vi "Controller Test Bench (17).vi"(5 "Folder to save file to":path=path "C:/Users/LAV-UFSC-2023/Documents/LAV-TCC/Dados-Experimentos/Dados-Bancada-LABVIEW", 6 "Signal Output\nControl":enum32{"White Noise", "Harmonic"}(tab), 7 "stop":bool, 8 "Enable Display":bool=TRUE, 9 "Accel. 2":bool, 10 "Output":bool=TRUE) -> (0 "New file path":path, 2 "Accel. 1 Raw":dbl[](graph), 3 "Output Signal":dynamicdata(graph))   [LabVIEW 2022 SP3]
uses:
  WhiteNoise.ctl
  <vilib>/Utility/error.llb/DialogType.ctl
  <vilib>/Platform/TimedLoop/XDataNode/timing_clust.ctl
  <vilib>/Platform/TimedLoop/XDataNode/nitl_modes.ctl
  <vilib>/Platform/TimedLoop/XDataNode/wakeup.ctl
  <vilib>/DAQmx/create/channels.llb/DAQmx Create Channel (AI-Acceleration-Accelerometer).vi
  <vilib>/DAQmx/configure/timing.llb/DAQmx Timing (Sample Clock).vi
  <vilib>/DAQmx/miscellaneous.llb/DAQmx Fill In Error Info.vi
  <vilib>/platform/TimedLoop/XDataNode/XDataNode.xnode
  <vilib>/DAQmx/read.llb/DAQmx Read (Analog 1D DBL 1Chan NSamp).vi
  <vilib>/DAQmx/write.llb/DAQmx Write (Analog 2D DBL NChan NSamp).vi
  <vilib>/DAQmx/create/channels.llb/DAQmx Create Channel (AO-Voltage-Basic).vi
  <vilib>/measure/NI_MABase.lvlib
  <vilib>/Platform/TimedLoop/XDataNode/XDNodeRunTimeDep.lvlib
panel:
  out "Frame 2 Duration":i64
  out "Frame 1 Duration":i64
  in  "White Noise\nParameters":T2={"Seed"=0.0, "Standard Deviation"=2.0, "Reset"=FALSE, "Iterator"=1.0, "Seed"=-1, "Lower Cut-Off"=5.0, "Upper Cut-Off"=350.0} {"Upper Cut-Off" min=5.0 max=350.0 step=10.0; "Lower Cut-Off" min=5.0 max=350.0 step=10.0; "Standard Deviation" min=0.001 max=3.0 step=0.05 format="%0.2p"}
  in  "Hamonic\nParameters":T3={"Waveform Type"=0, "Frequency"=10.0, "Amplitude"=0.25} {"Frequency" min=5.0 max=350.0 step=10.0 format="%0.2p"; "Waveform Type" items=["Sine Wave", "Triangle Wave", "Square Wave", "Sawtooth Wave"]; "Amplitude" min=0.001 max=0.3 step=0.05 format="%0.2p"}
  # "Filter"
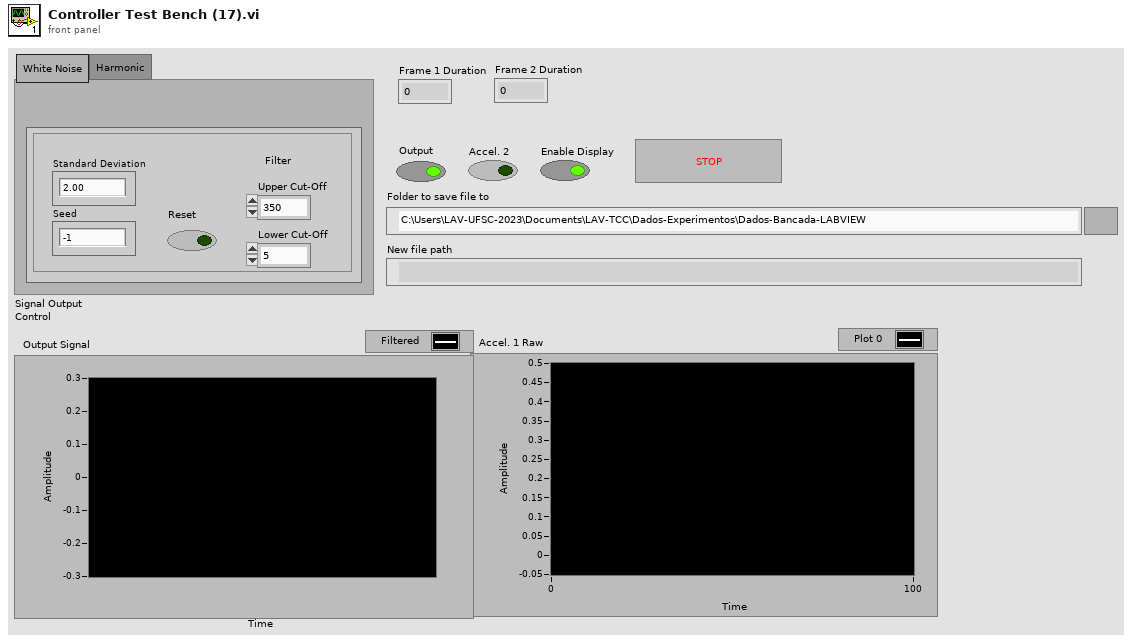
[diagram p1: front panel]
types:
  T1 = typedef "WhiteNoise.ctl" = dbl
  T2 = cluster{"Seed":T1, "Standard Deviation":dbl, "Reset":bool, "Iterator":dbl, "Seed":i8, "Lower Cut-Off":dbl, "Upper Cut-Off":dbl}
  T3 = cluster{"Waveform Type":u16, "Frequency":dbl, "Amplitude":dbl}
  T4 = typedef "DialogType.ctl" = u16
  T5 = enum16{"open", "open or create", "create or replace", "create", "open (read-only)"}
  T6 = typedef "XDNodeRunTimeDep.lvlib/timing_clust.ctl" = cluster{"Expected End [f-1]":u64, "Actual End [f-1]":u64, "Finished Late? [f-1]":bool, "Expected End [i-1]":u64, "Actual End [i-1]":u64, "Finished Late? [i-1]":bool, "Expected Start [i]":u64, "Actual Start [i]":u64, "Expected Start [f]":u64, "Actual Start [f]":u64, "Source Name":string, "Structure Name":string, "Period":i64, "Deadline":i64, "Offset":i64, "Start":i64, "Priority":i32, "Timeout":i32, "Mode":T7, "Wakeup Reason":T8, "Error":errorcluster, "Source Type":string, "Secondary Source Type":string, "Global End Time":u64, "Global Start Time":u64, "Frame Duration":u64, "Iteration Duration":u64, "Assigned CPU":i32, "I/O Scan Engine Mode":u32}
  T7 = typedef "XDNodeRunTimeDep.lvlib/nitl_modes.ctl" = enum32{"No Change", "Process missed periods, maintain original phase", "Discard missed periods, maintain original phase", "Process missed periods, ignore original phase", "Discard missed periods, ignore original phase"}
  T8 = typedef "XDNodeRunTimeDep.lvlib/wakeup.ctl" = enum32{"Normal", "Aborted", "Asynchronous wakeup", "Timing source error", "Timed loop error", "Timeout"}
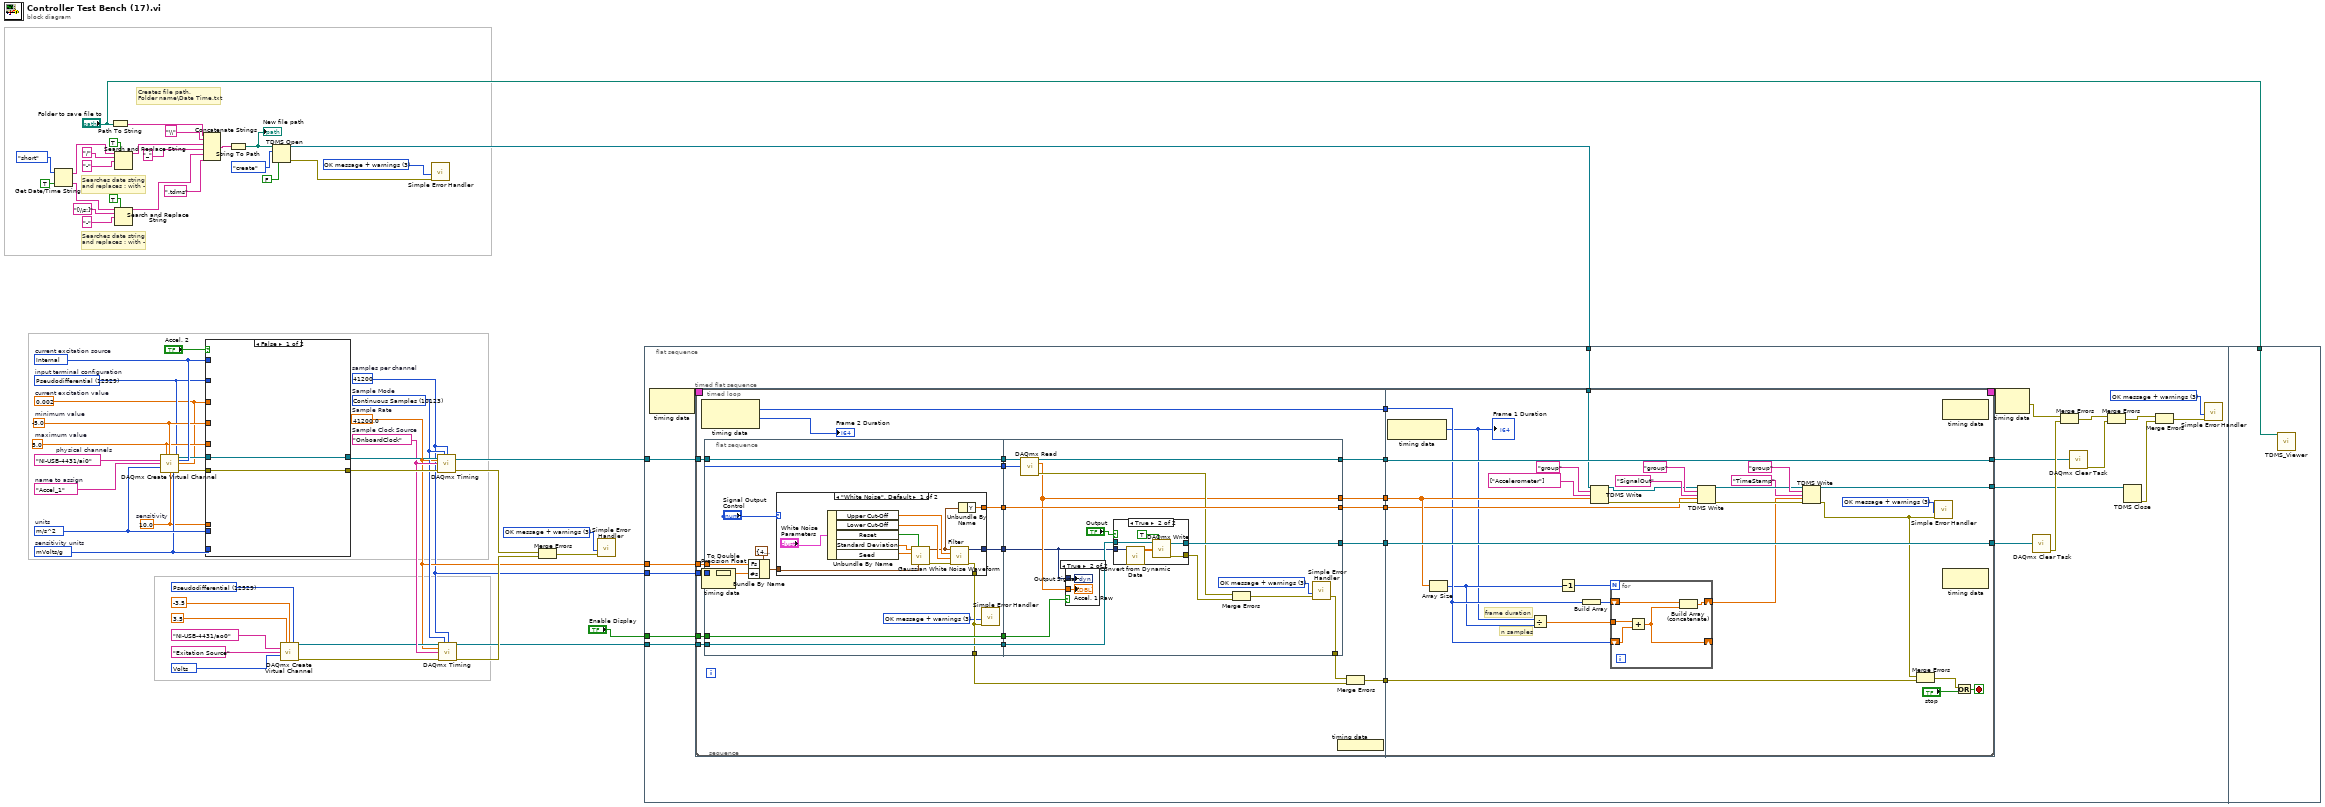
[diagram p0: block diagram]
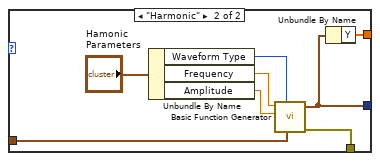
[diagram p2: hidden frame]
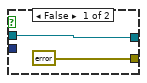
[diagram p4: hidden frame]
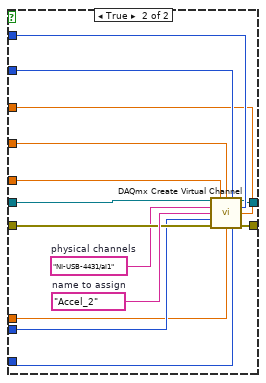
[diagram p5: hidden frame]
diagram:
  w10 = T4 3 items=["no dialog", "OK message", "continue or stop message", "OK message + warnings", "continue/stop + warnings"] ("type of dialog (OK msg:1)")
  w6 = 41200  # samples per channel
  w12 = T4 3 items=["no dialog", "OK message", "continue or stop message", "OK message + warnings", "continue/stop + warnings"] ("type of dialog (OK msg:1)")
  w45 = 12529 items=["Default"=-1, "RSE"=10083, "Differential"=10106, "Pseudodifferential"=12529] ("output terminal configuration")
  w43 = 10348 items=["Volts"=10348, "From Custom Scale"=10065] ("units")
  w49 = 12509 items=["mVolts/g"=12509, "Volts/g"=12510]  # sensitivity units
  w40 = 10.0  # sensitivity
  w48 = 0.002  # current excitation value
  w56 = 10200 items=["Internal"=10200, "External"=10167, "None"=10230]  # current excitation source
  w50 = tag "NI-USB-4431/ai0"  # physical channels
  w37 = tag "OnboardClock"  # Sample Clock Source
  w7 = 41200.0  # Sample Rate
  w36 = 10123 items=["Finite Samples"=10178, "Continuous Samples"=10123, "Hardware Timed Single Point"=12522]  # Sample Mode
  w52 = 12529 items=["default"=-1, "RSE"=10083, "NRSE"=10078, "Differential"=10106, "Pseudodifferential"=12529]  # input terminal configuration
  w55 = -5.0  # minimum value
  w54 = 5.0  # maximum value
  w58 = "Accel_1"  # name to assign
  w53 = 12470 items=["g"=10186, "m/s^2"=12470, "in/s^2"=12471, "From Custom Scale"=10065]  # units
  # "Searches date string\nand replaces : with -"
  # "Searches date string\nand replaces : with -"
  # "Creates file path.\nFolder name\\Date Time.txt"
  n1 = Get Date/Time String(date format (0)=enum16{"short", "long", "abbreviated"}."short", want seconds? (F)=TRUE) -> (date string=w15:string, time string=w28:string)  [unwired: 1 in]
  n2 = Path To String(path="Folder to save file to") -> (string=w23:string)
  n3 = Search and Replace String(replace all?=TRUE ("replace all? (F)"), input string=w15, search string="/" ("replace string (\"\")"), replace string="-" ("replace string (\"\")")) -> (result string=w14:string)  [unwired: 4 in, 3 out]
  n4 = Search and Replace String(replace all?=TRUE ("replace all? (F)"), input string=w28, search string="[\\s:]" ("replace string (\"\")"), replace string="-" ("replace string (\"\")")) -> (result string=w21:string)  [unwired: 4 in, 3 out]
  n5 = call-poly <vilib>:"DAQmx Create Virtual Channel.vi"("maximum value"=w54, "minimum value"=w55, "input terminal configuration"=w52, "physical channels"=w50, "current excitation source"=w56, "name to assign"=w58, "current excitation value"=w48, "units"=w53, "sensitivity"=w40, "sensitivity units"=w49) -> ("task out"=w51:refnum<k21>, "error out"=w57:errorcluster)  [unwired: 4 in]
  n6 = Concatenate Strings(w23, "\\" ("string"), w14, "_" ("string"), w21, ".tdms" ("string")) -> (w19:string)
  n7 = case shown="False" "Accel. 2" {
    tunnel: w57 -> [w60 w73]
    tunnel: w56 -> [_ w72]
    tunnel: w55 -> [_ w71]
    tunnel: w54 -> [_ w70]
    tunnel: w53 -> [_ w69]
    tunnel: w52 -> [_ w68]
    tunnel: w51 -> [w59 w67]
    tunnel: w49 -> [_ w65]
    tunnel: w48 -> [_ w64]
    tunnel: w40 -> [_ w63]
    tunnel: [w60 w62] -> w39
    tunnel: [w59 w61] -> w38
    frame False {
    }
    frame True {
      w66 = tag "NI-USB-4431/ai1"  # physical channels
      w74 = "Accel_2"  # name to assign
      n8 = call-poly <vilib>:"DAQmx Create Virtual Channel.vi"("task in"=w67, "maximum value"=w70, "minimum value"=w71, "input terminal configuration"=w68, "physical channels"=w66, "current excitation source"=w72, "name to assign"=w74, "current excitation value"=w64, "units"=w69, "error in"=w73, "sensitivity"=w63, "sensitivity units"=w65) -> ("task out"=w61:refnum<k21>, "error out"=w62:errorcluster)  [unwired: 2 in]
    }
  }
  n9 = String To Path(string=w19) -> (path=w5:path)
  "New file path" <- w5
  n10 = TDMS Open(6:FALSE ("enable asynchronous? (T)"), 10:T5."create" ("operation (0:open)"), 11:w5) -> (0:w1:errorcluster, 3:w2:refnum<k34>)  [unwired: 4 in]
  n11 = call-poly <vilib>:"DAQmx Create Virtual Channel.vi"("maximum value"=3.5, "minimum value"=-3.5, "output terminal configuration"=w45, "physical channels"=tag "NI-USB-4431/ao0", "name to assign"="Exitation Source", "units"=w43) -> ("task out"=w34:refnum<k21>, "error out"=w35:errorcluster)  [unwired: 8 in]
  n12 = call <vilib>:"Simple Error Handler.vi"("type of dialog (OK msg:1)"=w12, "error in (no error)"=w1) -> ()  [unwired: 3 in, 5 out]
  n13 = call-poly <vilib>:"DAQmx Timing.vi"("task/channels in"=w38, "sample mode"=w36, "samples per channel"=w6, "rate"=w7, "source"=w37, "error in"=w39) -> ("task out"=w9:refnum<k21>, "error out"=w42:errorcluster)  [unwired: 8 in]
  n14 = call-poly <vilib>:"DAQmx Timing.vi"("task/channels in"=w34, "sample mode"=w36, "samples per channel"=w6, "rate"=w7, "source"=w37, "error in"=w35) -> ("task out"=w32:refnum<k21>, "error out"=w33:errorcluster)  [unwired: 8 in]
  n15 = Merge Errors(w42, w33) -> (w8:errorcluster)
  n16 = call <vilib>:"Simple Error Handler.vi"("type of dialog (OK msg:1)"=w10, "error in (no error)"=w8) -> ()  [unwired: 3 in, 5 out]
  n17 = flat-sequence {
    tunnel: w6 -> [w78]
    tunnel: w7 -> [w79]
    tunnel: "Enable Display" -> [w87]
    tunnel: w2 -> [w80]
    tunnel: w9 -> [w88]
    tunnel: w32 -> [w90]
    tunnel: "Folder to save file to" -> [w241]
    frame #0 {
      w91 = T4 3 items=["no dialog", "OK message", "continue or stop message", "OK message + warnings", "continue/stop + warnings"] ("type of dialog (OK msg:1)")
      n18 = node-c288() -> (w93:T6)  [unwired: 1 in]
      n19 = timed-loop {
        tunnel: w90 -> [w102]
        tunnel: [w101] -> w89
        tunnel: w88 -> [w100]
        tunnel: [w96] -> w85
        tunnel: [w94] -> w77
        tunnel: w87 -> [w99]
        tunnel: w78 -> [w98]
        timing: w93 -> [_]
        timing-out: [_] -> w92
        tunnel: w80 -> [w97]
        tunnel: w79 -> [w95]
        stop <- w223 stop-if-true
        n20 = timed-sequence {
          timing: _ -> [_]
          timing-out: _ -> [_]
          tunnel: w102 -> [w117]
          tunnel: [w116] -> w101
          tunnel: w100 -> [w115]
          tunnel: w99 -> [w114]
          tunnel: w98 -> [w113]
          tunnel: w97 -> [w109]
          tunnel: [w108] -> w96
          tunnel: w95 -> [w105]
          tunnel: [w104] -> w94
          n21 = timed-flat-sequence {
            tunnel: w117 -> [w131]
            tunnel: w115 -> [w130]
            tunnel: w114 -> [w127]
            tunnel: w113 -> [w126]
            tunnel: [w129] -> w112
            tunnel: [w128] -> w111
            tunnel: [w123] -> w110
            tunnel: [w122] -> w107
            tunnel: [w121] -> w106
            tunnel: w105 -> [w120]
            tunnel: [w119] -> w103
            tunnel: [w227] -> w116
            tunnel: w112 -> [w227]
            tunnel: w111 -> [w221]
            tunnel: w110 -> [w224]
            tunnel: w109 -> [w210]
            tunnel: [w221] -> w108
            tunnel: w107 -> [w219]
            tunnel: w106 -> [w211]
            tunnel: [w215] -> w104
            tunnel: w103 -> [w204]
            frame #0 {
              n22 = node-c288() -> (w119:i64, →"Frame 2 Duration":i64)  [unwired: 1 in]
              n23 = flat-sequence {
                tunnel: [w151] -> w137
                tunnel: [w147] -> w136
                tunnel: [w150] -> w135
                tunnel: [w148] -> w134
                tunnel: [w149] -> w133
                tunnel: [w143] -> w132
                tunnel: [w146] -> w124
                tunnel: w131 -> [w150]
                tunnel: w130 -> [w151]
                tunnel: w127 -> [w148]
                tunnel: w126 -> [w143]
                tunnel: w120 -> [w144]
                tunnel: w137 -> [w181]
                tunnel: w136 -> [w188]
                tunnel: w135 -> [w186]
                tunnel: w134 -> [w182]
                tunnel: w133 -> [w175]
                tunnel: w132 -> [w180]
                tunnel: [w176] -> w125
                tunnel: [w179] -> w122
                tunnel: [w188] -> w121
                tunnel: [w185] -> w129
                tunnel: [w183] -> w128
                frame #0 {
                  w145 = T4 3 items=["no dialog", "OK message", "continue or stop message", "OK message + warnings", "continue/stop + warnings"] ("type of dialog (OK msg:1)")
                  n24 = To Double Precision Float(number=w143) -> (double precision float=w142:dbl)
                  n25 = Bundle By Name(cluster=cluster{"Fs":dbl, "#s":dbl} {"Fs"=41200.0, "#s"=41200.0} ("sampling info"), "Fs"=w144, "#s"=w142) -> (w153:cluster{"Fs":dbl, "#s":dbl})
                  n26 = case shown="\"White Noise\", Default" "Signal Output\nControl" {
                    tunnel: w153 -> [w164 w173]
                    tunnel: [w157 w169] -> w149
                    tunnel: [w156 w168] -> w147
                    tunnel: [w155 w167] -> w146
                    frame "White Noise", Default {
                      n27 = Unbundle By Name("White Noise\nParameters") -> ("Upper Cut-Off"=w160:dbl, "Lower Cut-Off"=w159:dbl, "Reset"=w161:bool, "Standard Deviation"=w162:dbl, "Seed"=w163:T1)
                      n28 = call <vilib>:"Gaussian White Noise Waveform.vi"("sampling info"=w164, "reset signal"=w161, "seed"=w163, "standard deviation"=w162) -> ("error out"=w166:errorcluster, "signal out"=w158:waveform(dbl))  [unwired: 6 in]
                      n29 = call "Filter"("error in (no error)"=w166, "Lower Cut-Off"=w159, "Upper Cut-Off"=w160, "Signal"=w158) -> ("error out"=w155:errorcluster, "Filtered Signal"=w157:dynamicdata)  [unwired: 6 in]
                      n30 = Unbundle By Name(w158) -> ("Y"=w156:dbl[])
                    }
                    frame "Harmonic" {
                      n31 = Unbundle By Name("Hamonic\nParameters") -> ("Waveform Type"=w172:u16, "Frequency"=w171:dbl, "Amplitude"=w170:dbl)
                      n32 = call <vilib>:"Basic Function Generator.vi"("sampling info"=w173, "signal type"=w172, "amplitude"=w170, "frequency"=w171) -> ("error out"=w167:errorcluster, "signal out"=w169:waveform(dbl))  [unwired: 5 in, 1 out]
                      n33 = Unbundle By Name(w169) -> ("Y"=w168:dbl[])
                    }
                  }
                  n34 = call <vilib>:"Simple Error Handler.vi"("type of dialog (OK msg:1)"=w145, "error in (no error)"=w146) -> ()  [unwired: 3 in, 5 out]
                }
                frame #1 {
                  w178 = T4 3 items=["no dialog", "OK message", "continue or stop message", "OK message + warnings", "continue/stop + warnings"] ("type of dialog (OK msg:1)")
                  n35 = call-poly <vilib>:"DAQmx Read.vi"("task/channels in"=w181, "number of samples per channel"=w180) -> ("task out"=w183:refnum<k21>, "data"=w179:dbl[], "error out"=w184:errorcluster)  [unwired: 11 in]
                  n36 = case shown="True" w182 {
                    tunnel: w179 -> [_ w190]
                    tunnel: w175 -> [_ w189]
                    frame False {
                    }
                    frame True {
                      "Accel. 1 Raw" <- w190
                      "Output Signal" <- w189
                    }
                  }
                  n37 = case shown="True" "Output" {
                    tunnel: w186 -> [w192 w198]
                    tunnel: [errorcluster {"status"=FALSE, "code"=0, "source"=""} ("error out") w196] -> w177
                    tunnel: [w192 w197] -> w185
                    tunnel: w175 -> [_ w195]
                    frame False {
                    }
                    frame True {
                      n38 = call "Convert from Dynamic Data"("Dynamic Data Type"=w195) -> ("Array"=w194:dbl[][])  [unwired: 3 in]
                      n39 = call-poly <vilib>:"DAQmx Write.vi"("task/channels in"=w198, "auto start"=TRUE, "data"=w194) -> ("task out"=w197:refnum<k21>, "error out"=w196:errorcluster)  [unwired: 10 in, 1 out]
                    }
                  }
                  n40 = Merge Errors(w184, w177) -> (w176:errorcluster)
                  n41 = call <vilib>:"Simple Error Handler.vi"("type of dialog (OK msg:1)"=w178, "error in (no error)"=w176) -> ()  [unwired: 3 in, 5 out]
                }
              }
              n42 = node-c288() -> ()  [unwired: 1 out]
              n43 = Merge Errors(w125, w124) -> (w123:errorcluster)
            }
            frame #1 {
              w222 = T4 3 items=["no dialog", "OK message", "continue or stop message", "OK message + warnings", "continue/stop + warnings"] ("type of dialog (OK msg:1)")
              # "n samples"
              # "frame duration"
              n44 = node-c288() -> (w199:i64)  [unwired: 1 in]
              "Frame 1 Duration" <- w199
              n45 = Array Size(array=w219) -> (size(s)=w203:i32)
              n46 = Divide(x=w199, y=w203) -> (x/y=w200:dbl)
              n47 = Decrement(x=w203) -> (x-1=w202:i32)
              n48 = Build Array(w204) -> (w201:i64[])
              n49 = TDMS Write(0:w210, 5:"group" ("group name in (Untitled)"), 7:string[] ["Accelerometer"] ("channel name(s) in (Untitled)"), 9:w219) -> (4:w209:refnum<k34>, 15:w213:errorcluster)  [unwired: 2 in, 2 out]
              n50 = for {
                N: w202 -> [_]
                shift-right: [w228] -> _
                shift-left: w204 -> [w232]
                tunnel: w200 -> [w231]
                shift-right: [w230] -> w205
                shift-left: w201 -> [w229]
                n51 = Add(x=w231, y=w232) -> (x+y=w228:dbl)
                n52 = Build Array (concatenate)(w229, w228) -> (w230:dbl[])
              }
              n53 = TDMS Write(0:w209, 5:"group" ("group name in (Untitled)"), 7:"SignalOut", 9:w211, 11:w213) -> (4:w208:refnum<k34>, 15:w212:errorcluster)  [unwired: 1 in, 2 out]
              n54 = TDMS Write(0:w208, 5:"group" ("group name in (Untitled)"), 7:"TimeStamp", 9:w205, 11:w212) -> (4:w215:refnum<k34>, 15:w207:errorcluster)  [unwired: 1 in, 2 out]
              n55 = Merge Errors(w207, w224) -> (w226:errorcluster)
              n56 = call <vilib>:"Simple Error Handler.vi"("type of dialog (OK msg:1)"=w222, "error in (no error)"=w207) -> ()  [unwired: 3 in, 5 out]
              n57 = node-c288() -> ()  [unwired: 1 in, 1 out]
              n58 = Or(x=w226, y="stop") -> (x .or. y?=w223:bool)
            }
          }
        }
        n59 = node-c288() -> ()  [unwired: 1 in, 1 out]
        n60 = node-c288() -> ()  [unwired: 1 in, 1 out]
      }
      n61 = node-c288(w92) -> (w81:errorcluster)
      n62 = call <vilib>:"DAQmx Clear Task.vi"("task in"=w89) -> ("error out"=w86:errorcluster)  [unwired: 14 in]
      n63 = Merge Errors(w81, w86) -> (w84:errorcluster)
      n64 = call <vilib>:"DAQmx Clear Task.vi"("task in"=w85) -> ("error out"=w83:errorcluster)  [unwired: 14 in]
      n65 = Merge Errors(w84, w83) -> (w76:errorcluster)
      n66 = TDMS Close(11:w77) -> (0:w75:errorcluster)  [unwired: 1 in, 1 out]
      n67 = Merge Errors(w76, w75) -> (w82:errorcluster)
      n68 = call <vilib>:"Simple Error Handler.vi"("type of dialog (OK msg:1)"=w91, "error in (no error)"=w82) -> ()  [unwired: 3 in, 5 out]
    }
    frame #1 {
      n69 = call "TDMS_Viewer.vi"("Data Directory"=w241) -> ()  [unwired: 11 in]
    }
  }
